vi "Configure Reading Buffer Data Characteristics.vi"(6 "Timestamp Resolution (1E-6 S)":dbl=1e-06, 7 "Enable Source Value (F: Disable)":bool, 8 "error in (no error)":errorcluster, 9 "Enable Timestamp (F: Disable)":bool, 10 "Reading Buffer (smua.nvbuffer1)":string="smua.nvbuffer1", 11 "VISA resource name":refnum<visa-resource-name>) -> (0 "error out":errorcluster, 3 "VISA resource name out":refnum<visa-resource-name>)   [LabVIEW 2020, in "Keithley 2600 Series.lvlib"]
doc: "Configures the basic settings of the reading buffer data.\n\n<b>Note:</b>\nThis VI also clears all readings from the specified buffer."
uses:
  <instrlib>/Keithley 2600 Series/Keithley 2600 Series.lvlib
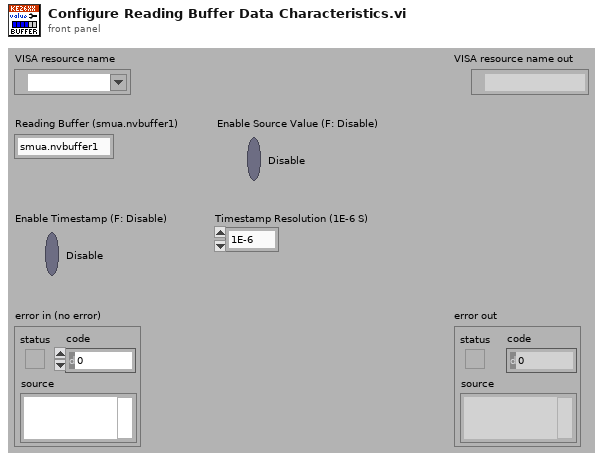
[diagram p1: front panel]
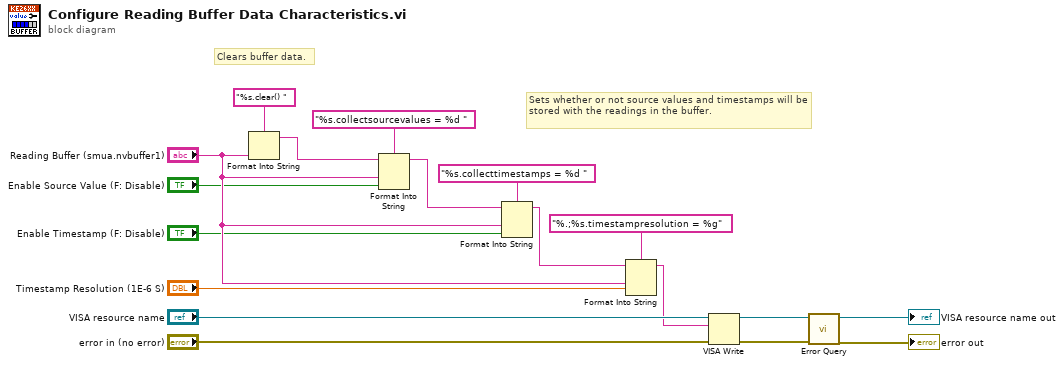
[diagram p0: block diagram]
diagram:
  # "Sets whether or not source values and timestamps will be stored with the readings in the buffer."
  # "Clears buffer data."
  n1 = Format Into String(format string="%s.clear() ", "Reading Buffer (smua.nvbuffer1)") -> (resulting string=w6:string)  [unwired: 2 in, 1 out]
  n2 = Format Into String(format string="%s.collectsourcevalues = %d ", initial string=w6, "Reading Buffer (smua.nvbuffer1)", "Enable Source Value (F: Disable)") -> (resulting string=w17:string)  [unwired: 1 in, 1 out]
  n3 = Format Into String(format string="%s.collecttimestamps = %d ", initial string=w17, "Reading Buffer (smua.nvbuffer1)", "Enable Timestamp (F: Disable)") -> (resulting string=w15:string)  [unwired: 1 in, 1 out]
  n4 = Format Into String(format string="%.;%s.timestampresolution = %g", initial string=w15, "Reading Buffer (smua.nvbuffer1)", "Timestamp Resolution (1E-6 S)") -> (resulting string=w5:string)  [unwired: 1 in, 1 out]
  n5 = VISA Write(VISA resource name="VISA resource name", write buffer=w5, error in (no error)="error in (no error)") -> (VISA resource name out=w10:refnum<visa-resource-name>, error out=w9:errorcluster)  [unwired: 1 out]
  n6 = call <instrlib>:"Error Query.vi"("error in (no error)"=w9, "VISA resource name"=w10) -> ("error out"=→"error out":errorcluster, "VISA resource name out"=→"VISA resource name out":refnum<visa-resource-name>)  [unwired: 6 in, 2 out]
